vi "Field_C switch mode.vi"(8 "error in (no error)":errorcluster, 9 "PSU Status":T8 {"Trip Current" format="%.3f"; "Trip Field" format="%.4f"; "Voltage" format="%.2f"; "Field Constant" format="%.6f"; "MID Setpoint (T)" format="%.4f"; "MID Setpoint (A)" format="%.3f"; "MAX Setpoint (T)" format="%.4f"; "MAX Setpoint (A)" format="%.3f"; "Heater Voltage" format="%.2f"; "V Limit (V)" format="%.2f"; "Ramp Rate (A/s)" format="%.3f"; "Output (A)" format="%.3f"; "Output (T)" format="%.4f"; "Persistent Current" format="%.3f"; "Persistent Field" format="%.4f"}, 10 "Overall status in":T3, 11 "Magnet Constants":T2) -> (0 "error out":errorcluster, 2 "PSU Status out":T8 {"Trip Current" format="%.3f"; "Trip Field" format="%.4f"; "Voltage" format="%.2f"; "Field Constant" format="%.6f"; "MID Setpoint (T)" format="%.4f"; "MID Setpoint (A)" format="%.3f"; "MAX Setpoint (T)" format="%.4f"; "MAX Setpoint (A)" format="%.3f"; "Heater Voltage" format="%.2f"; "V Limit (V)" format="%.2f"; "Ramp Rate (A/s)" format="%.3f"; "Output (A)" format="%.3f"; "Output (T)" format="%.4f"; "Persistent Current" format="%.3f"; "Persistent Field" format="%.4f"}, 3 "Overall status out":T3)   [LabVIEW 2024, in "Magnet module.lvlib"]
uses:
  Magnet module.lvlib
  ctl/Overall status.ctl
  ctl/SetField data.ctl
  ctl/Magnet mode public.ctl
  ctl/Actual magnet state.ctl
  ctl/Magnet mode.ctl
  ctl/RampingOutput.ctl
  <instrlib>/SMS drivers/Public/PSU Status.ctl
  ctl/Magnet config constants.ctl
  <instrlib>/SMS drivers/Cryogenic Ltd SMSXXX.lvlib
panel:
  out "Heater switched":bool
  in  "Desired.Mode":T1
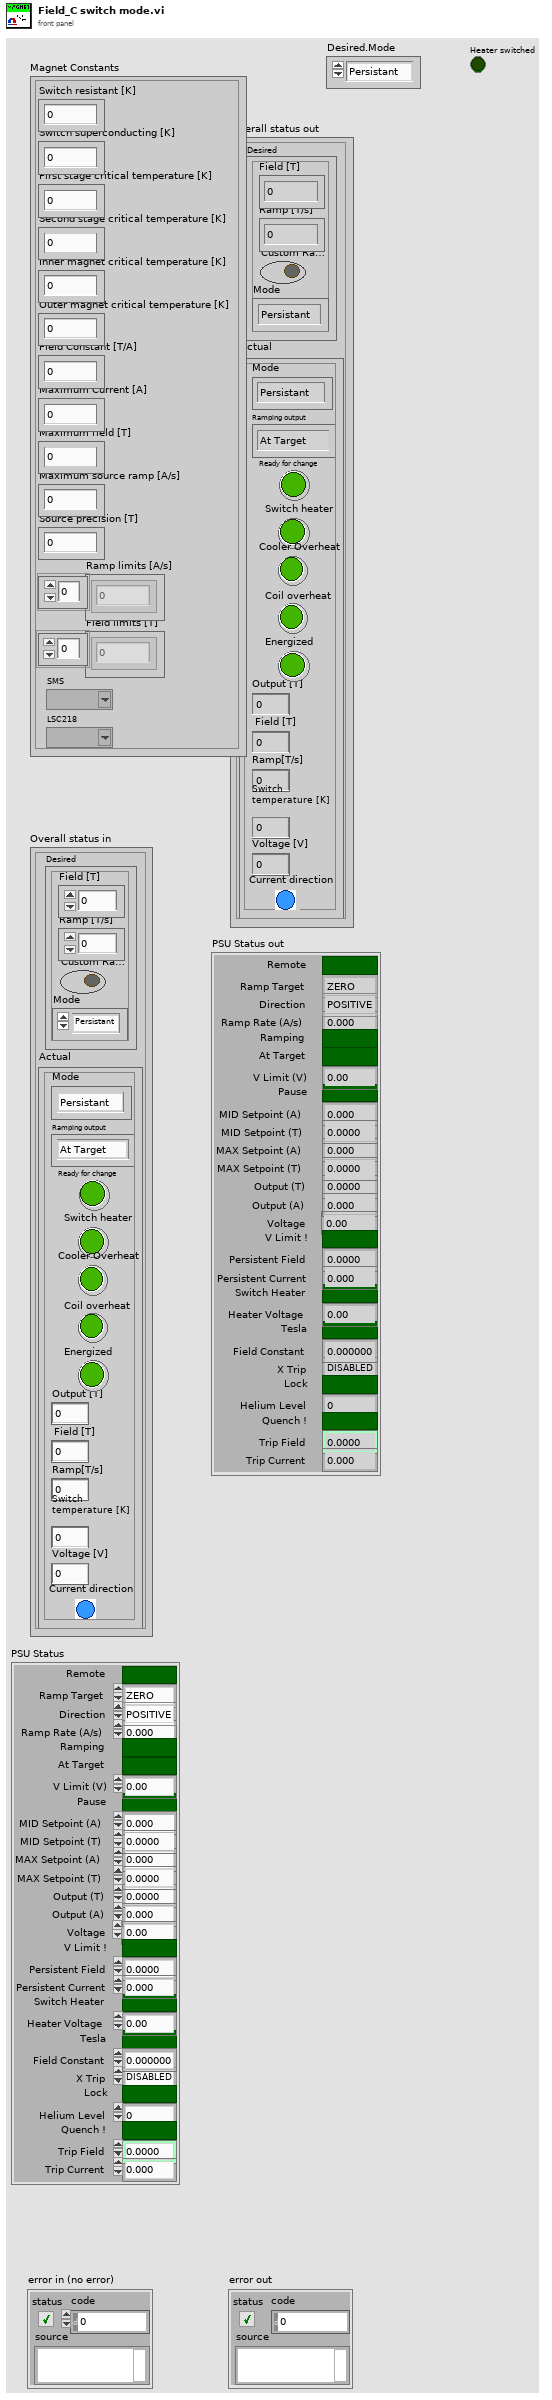
[diagram p1: front panel]
types:
  T1 = typedef "Magnet module.lvlib/Magnet mode public.ctl" = enum16{"Persistant", "Ramping"}
  T2 = typedef "Magnet module.lvlib/Magnet config constants.ctl" = cluster{"Switch resistant [K]":dbl, "Switch superconducting [K]":dbl, "First stage critical temperature [K]":dbl, "Second stage critical temperature [K]":dbl, "Inner magnet critical temperature [K]":dbl, "Outer magnet critical temperature [K]":dbl, "Field Constant [T/A]":dbl, "Maximum Current [A]":dbl, "Maximum field [T]":dbl, "Maximum source ramp [A/s]":dbl, "Source precision [T]":dbl, "Ramp limits [A/s]":dbl[], "Field limits [T]":dbl[], "SMS":refnum<visa-resource-name>, "LSC218":refnum<visa-resource-name>}
  T3 = typedef "Magnet module.lvlib/Overall status.ctl" = cluster{"Desired":T4, "Actual":T5}
  T4 = typedef "Magnet module.lvlib/SetField data.ctl" = cluster{"Field [T]":dbl, "Ramp [T/s]":dbl, "Custom Ramp?":bool, "Mode":T1}
  T5 = typedef "Magnet module.lvlib/Actual magnet state.ctl" = cluster{"Mode":T6, "Ramping output":T7, "Ready for change":bool, "Switch heater":bool, "Cooler Overheat":bool, "Coil overheat":bool, "Energized":bool, "Output [T]":dbl, "Field [T]":dbl, "Ramp[T/s]":dbl, "Switch\ntemperature [K]":dbl, "Voltage [V]":dbl, "Current direction":bool}
  T6 = typedef "Magnet module.lvlib/Magnet mode.ctl" = enum16{"Persistant", "Switching", "Ramping", "Quenched"}
  T7 = typedef "Magnet module.lvlib/RampingOutput.ctl" = enum16{"At Target", "Go up", "Go down"}
  T8 = typedef "Cryogenic Ltd SMSXXX.lvlib/PSU Status.ctl" = cluster{"Ramp Target":enum16{"ZERO", "MID", "MAX"}, "Pause":bool, "Switch Heater":bool, "Persistent Field":dbl, "Persistent Current":dbl, "Tesla":bool, "Output (T)":dbl, "Output (A)":dbl, "X Trip":enum16{"DISABLED", "ENABLED", "ACTIVE"}, "Ramp Rate (A/s)":dbl, "V Limit (V)":dbl, "Heater Voltage":dbl, "MAX Setpoint (A)":dbl, "MAX Setpoint (T)":dbl, "MID Setpoint (A)":dbl, "MID Setpoint (T)":dbl, "Lock":bool, "Field Constant":dbl, "Remote":bool, "Direction":enum16{"POSITIVE", "NEGATIVE", "OPEN", "UNIPOLAR"}, "Helium Level":u16, "Quench !":bool, "Voltage":dbl, "V Limit !":bool, "Ramping":bool, "At Target":bool, "Trip Field":dbl, "Trip Current":dbl}
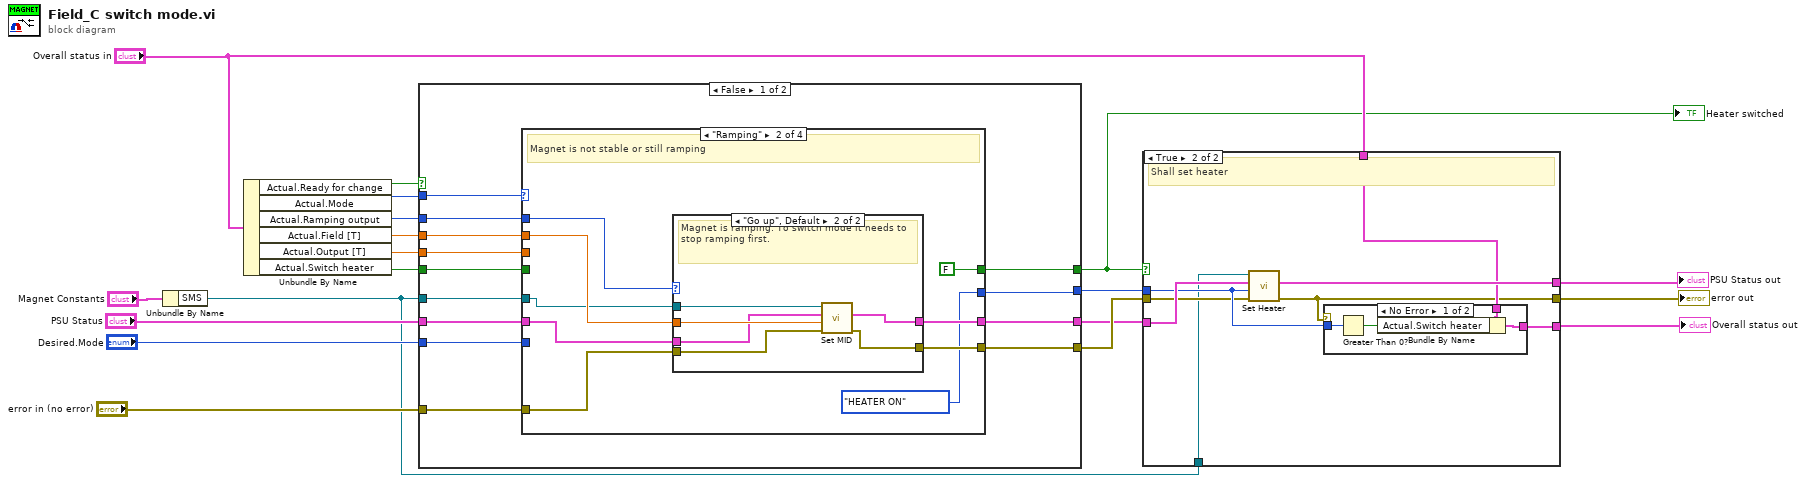
[diagram p0: block diagram]
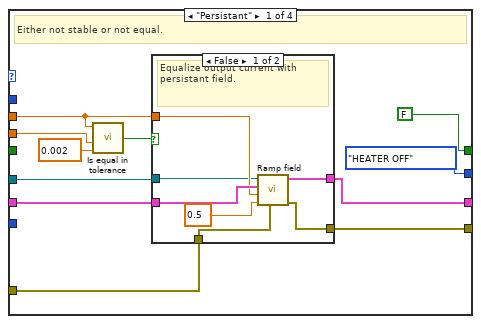
[diagram p4: hidden frame]
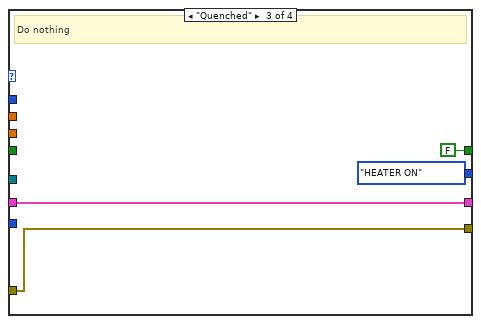
[diagram p7: hidden frame]
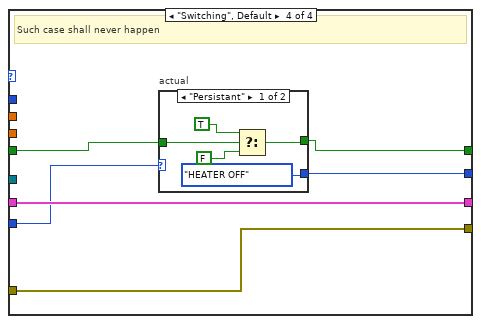
[diagram p8: hidden frame]
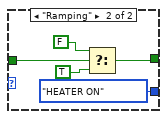
[diagram p9: hidden frame]
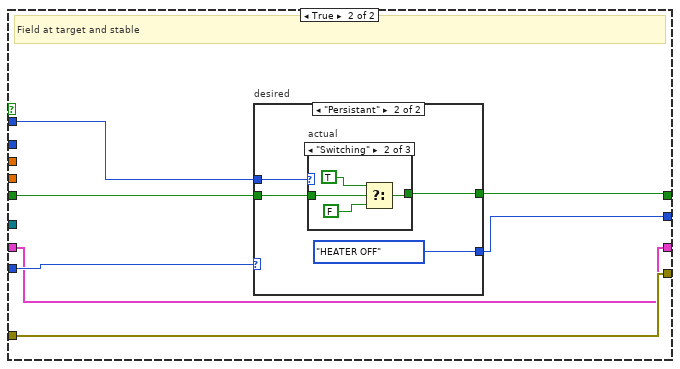
[diagram p10: hidden frame]
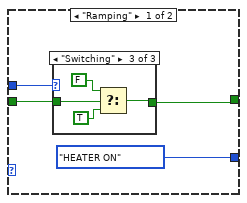
[diagram p11: hidden frame]
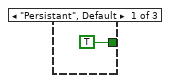
[diagram p12: hidden frame]
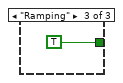
[diagram p15: hidden frame]
diagram:
  n1 = Unbundle By Name("Magnet Constants") -> ("SMS"=w1:refnum<visa-resource-name>)
  n2 = Unbundle By Name("Overall status in") -> ("Actual.Ready for change"=w17:bool, "Actual.Mode"=w19:T6, "Actual.Ramping output"=w15:T7, "Actual.Field [T]"=w14:dbl, "Actual.Output [T]"=w12:dbl, "Actual.Switch heater"=w11:bool)
  n3 = case shown="False" w17 {
    tunnel: "Desired.Mode" -> [w23 w92]
    tunnel: w1 -> [w25 _]
    tunnel: "PSU Status" -> [w29 w90]
    tunnel: w19 -> [w32 w96]
    tunnel: [w27 w91] -> w5
    tunnel: w15 -> [w31 _]
    tunnel: w14 -> [w30 _]
    tunnel: "error in (no error)" -> [w28 w91]
    tunnel: w12 -> [w26 _]
    tunnel: w11 -> [w22 w95]
    tunnel: [w20 w94] -> w2
    tunnel: [w21 w93] -> w10
    tunnel: [w24 w90] -> w3
    frame False {
      n4 = case shown="\"Ramping\"" w32 {
        tunnel: w31 -> [_ w61 _ _]
        tunnel: w30 -> [w40 w60 _ _]
        tunnel: w29 -> [w39 w59 w73 w78]
        tunnel: w28 -> [w35 w58 w72 w79]
        tunnel: [w36 w57 w72 w79] -> w27
        tunnel: [w38 w56 w73 w78] -> w24
        tunnel: w26 -> [w42 _ _ _]
        tunnel: w25 -> [w37 w55 _ _]
        tunnel: w23 -> [_ _ _ w77]
        tunnel: w22 -> [_ _ _ w76]
        tunnel: [enum16{"HEATER OFF", "HEATER ON"}."HEATER OFF" ("Heater (On/Off)") enum16{"HEATER OFF", "HEATER ON"}."HEATER ON" ("Heater (On/Off)") enum16{"HEATER OFF", "HEATER ON"}."HEATER ON" ("Heater (On/Off)") w75] -> w21
        tunnel: [FALSE ("f") FALSE ("f") FALSE ("f") w74] -> w20
        frame "Persistant" {
          # "Either not stable or not equal."
          n5 = call "Is equal in tolerance.vi"("Absolut tolerance"=0.002, "Reference value"=w42, "Input value"=w40) -> ("Is in range"=w41:bool)  [unwired: 1 in]
          n6 = case shown="False" w41 {
            tunnel: w40 -> [w48 _]
            tunnel: w39 -> [w50 w52]
            tunnel: [w47 w52] -> w38
            tunnel: w37 -> [w46 _]
            tunnel: [w45 w51] -> w36
            tunnel: w35 -> [w44 w51]
            frame False {
              # "Equalize output current with persistant field."
              n7 = call "Ramp field.vi"("Error In"=w44, "Ramp to set [A/s]"=0.5, "Field to set [T]"=w48, "PSU Status In"=w50, "VISA Refnum in"=w46) -> ("error out"=w45:errorcluster, "PSU Status Out"=w47:T8)  [unwired: 3 in, 2 out]
            }
            frame True {
              # "They are equal, but probably not stable."
            }
          }
        }
        frame "Ramping" {
          # "Magnet is not stable or still ramping"
          n8 = case shown="\"Go up\", Default" w61 {
            tunnel: w60 -> [_ w69]
            tunnel: w59 -> [w62 w68]
            tunnel: w55 -> [_ w64]
            tunnel: w58 -> [w63 w67]
            tunnel: [w63 w66] -> w57
            tunnel: [w62 w65] -> w56
            frame "At Target" {
              # "Do nothing, just wait till field stabilize"
              # "Just come to target"
            }
            frame "Go up", Default {
              # "Magnet is ramping. To switch mode it needs to stop ramping first."
              n9 = call <instrlib>:"Set MID.vi"("Error in (no error)"=w67, "MID (T or A)"=w69, "PSU Status In"=w68, "VISA Resource Name In"=w64) -> ("Error out"=w66:errorcluster, "PSU Status Out"=w65:T8)  [unwired: 4 in, 2 out]
            }
          }
        }
        frame "Quenched" {
          # "Do nothing"
        }
        frame "Switching", Default {
          # "Such case shall never happen"
          n10 = case "actual" shown="\"Persistant\"" w77 {
            tunnel: [w81 w86] -> w74
            tunnel: w76 -> [w84 w89]
            tunnel: [enum16{"HEATER OFF", "HEATER ON"}."HEATER OFF" ("Heater (On/Off)") enum16{"HEATER OFF", "HEATER ON"}."HEATER ON" ("Heater (On/Off)")] -> w75
            frame "Persistant" {
              n11 = Select(t=TRUE, s=w84, f=FALSE) -> (s? t:f=w81:bool)
            }
            frame "Ramping" {
              n12 = Select(t=FALSE, s=w89, f=TRUE) -> (s? t:f=w86:bool)
            }
          }
        }
      }
    }
    frame True {
      # "Field at target and stable"
      n13 = case "desired" shown="\"Persistant\"" w92 {
        tunnel: [enum16{"HEATER OFF", "HEATER ON"}."HEATER ON" ("Heater (On/Off)") enum16{"HEATER OFF", "HEATER ON"}."HEATER OFF" ("Heater (On/Off)")] -> w93
        tunnel: w96 -> [w100 w108]
        tunnel: [w98 w107] -> w94
        tunnel: w95 -> [w99 w106]
        frame "Ramping" {
          n14 = case shown="\"Switching\"" w100 {
            tunnel: w99 -> [_ _ w105]
            tunnel: [TRUE ("f") _ w102] -> w98
            frame "Persistant", Default {
            }
            frame "Ramping" {
            }
            frame "Switching" {
              n15 = Select(t=FALSE ("Switch heater"), s=w105, f=TRUE) -> (s? t:f=w102:bool)
            }
          }
        }
        frame "Persistant" {
          n16 = case "actual" shown="\"Switching\"" w108 {
            tunnel: [_ w110 TRUE] -> w107
            tunnel: w106 -> [_ w113 _]
            frame "Persistant", Default {
            }
            frame "Switching" {
              n17 = Select(t=TRUE, s=w113, f=FALSE) -> (s? t:f=w110:bool)
            }
            frame "Ramping" {
            }
          }
        }
      }
    }
  }
  "Heater switched" <- w2
  n18 = case shown="True" w2 {
    tunnel: w10 -> [_ w123]
    tunnel: [w116 w125] -> w9
    tunnel: w3 -> [w116 w124]
    tunnel: [w115 w118] -> w8
    tunnel: "Overall status in" -> [w117 w122]
    tunnel: [w117 w121] -> w6
    tunnel: w5 -> [w115 w120]
    tunnel: w1 -> [_ w119]
    frame False {
      # "No need to set heater"
    }
    frame True {
      # "Shall set heater"
      n19 = call <instrlib>:"Set Heater.vi"("Error in (no error)"=w120, "Heater (On/Off)"=w123, "PSU Status In"=w124, "VISA Resource Name In"=w119) -> ("Error out"=w118:errorcluster, "PSU Status Out"=w125:T8)  [unwired: 4 in, 2 out]
      n20 = case shown="No Error" w118 {
        tunnel: w123 -> [w129 _]
        tunnel: w122 -> [w128 w130]
        tunnel: [w127 w130] -> w121
        frame No Error {
          n21 = Greater Than 0?(x=w129) -> (x > 0?=w126:bool)
          n22 = Bundle By Name(cluster=w128, "Actual.Switch heater"=w126) -> (w127:T3)
        }
        frame Error {
        }
      }
    }
  }
  "Overall status out" <- w6
  "error out" <- w8
  "PSU Status out" <- w9
